vi "First Step Validation FFT.vi"(5 "FFT Array":dbl[](array[numeric]), 6 "Threshold Amp":dbl, 7 "Max Delta Difference % between bins":dbl=1.0, 8 "Windowing":T1(ring), 9 "Last Discard Bins":i32=255, 10 "Init Discard Bins":i32=10, 11 "#Signals":i32) -> (1 "Array check delta amp":bool[](array[boolean]), 2 "Array Check amp":bool[](array[boolean]), 3 "Inter Freq Array":dbl[](array[numeric]))   [LabVIEW 2014]
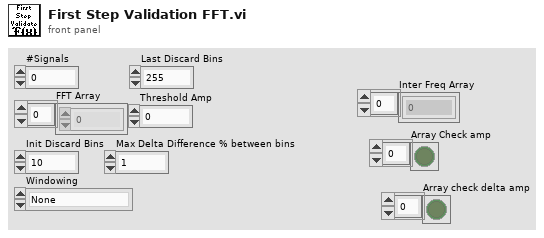
[diagram p1: front panel]
types:
  T1 = enum16{"None", "Hanning", "Hamming", "Blackman", "Blackman-Harris"}
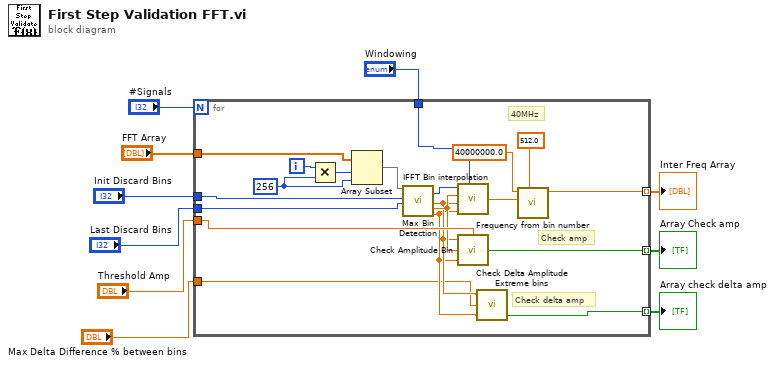
[diagram p0: block diagram]
diagram:
  n1 = for {
    N: "#Signals" -> [_]
    tunnel: "FFT Array" -> [w30]
    tunnel: "Init Discard Bins" -> [w25]
    tunnel: "Last Discard Bins" -> [w24]
    tunnel: "Threshold Amp" -> [w22]
    tunnel: [w20] -> w2 mode=indexing
    tunnel: "Max Delta Difference % between bins" -> [w12]
    tunnel: [w11] -> w1 mode=indexing
    tunnel: "Windowing" -> [w16]
    tunnel: [w15] -> w3 mode=indexing
    i -> [w29]
    w27 = 256 ("y")
    # "Check amp"
    # "Check delta amp"
    # "40MHz"
    n2 = Multiply(x=w29, y=w27) -> (x*y=w28:i32)
    n3 = Array Subset(array=w30, index=w28, length=w27) -> (w26:dbl[])
    n4 = call "Max Bin Detection.vi"("FFT Array"=w26, "Init Discard Bins"=w25, "Last Discard Bins"=w24) -> ("Max Bin"=w23:i32, "Prev Max Amp"=w14:dbl, "Max Amp"=w21:dbl, "Succ Max Amp"=w13:dbl)  [unwired: 11 in, 2 out]
    n5 = call "IFFT Bin interpolation.vi"("Max Bin"=w23, "Max Amp"=w21, "Prev Max Amp"=w14, "Succ Max Amp"=w13, "Windowing"=w16) -> ("Interpolate Bin"=w19:dbl)
    n6 = call "Check Amplitude Bin.vi"("Threshold Amp"=w22, "Succ Max Amp"=w13, "Max Amp"=w21, "Prev Max Amp"=w14) -> ("Check Amp Ok?"=w20:bool)
    n7 = call "Check Delta Amplitude Extreme bins.vi"("Succ Max Amp"=w13, "Max Difference %"=w12, "Prev Max Amp"=w14) -> ("Check Delta Amp Ok?"=w11:bool)  [unwired: 1 in, 1 out]
    n8 = call "Frequency from bin number.vi"("FFT size"=512.0, "Bin number"=w19, "Sample Rate (S/s)"=40000000.0) -> ("Detected Frequency (Hz)"=w15:dbl)  [unwired: 8 in]
  }
  "Inter Freq Array" <- w3
  "Array Check amp" <- w2
  "Array check delta amp" <- w1
